vi "DAQ Assist.vi"(4 "timeout (s)":dbl=10.0 format="%0.2f", 5 "error in":errorcluster, 7 "stop (F)":bool, 10 "device name":tag="Mantis1_1Mod4") -> (14 "task out":refnum<k21>, 15 "data":dynamicdata(waveform), 18 "stopped":bool, 19 "error out":errorcluster)   [LabVIEW 2015]
doc: "Creates, edits, and runs tasks using NI-DAQmx. Refer to the NI-DAQmx Readme for a complete listing of devices NI-DAQmx supports.\n\nWhen you place this Express VI on the block diagram, the DAQ Assistant launches to create a new task. After you create a task, you can double-click the DAQ Assistant Express VI to edit that task. For continuous measurement or generation, place a while loop around the DAQ Assistant Express VI."
uses:
  <vilib>/DAQmx/read.llb/DAQmx Read.vi
  <vilib>/DAQmx/read.llb/DAQmx Read (Counter 1D U32 NChan 1Samp).vi
  <vilib>/DAQmx/miscellaneous.llb/DAQmx Fill In Error Info.vi
  <vilib>/DAQmx/create/channels.llb/DAQmx Create Channel (CI-Count Edges).vi
  <resource>/objmgr/daqmx.rc
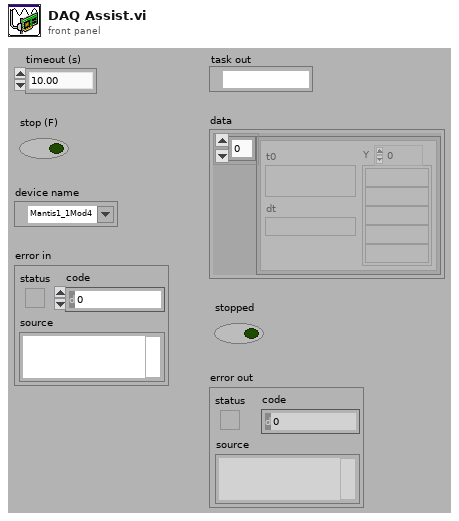
[diagram p1: front panel]
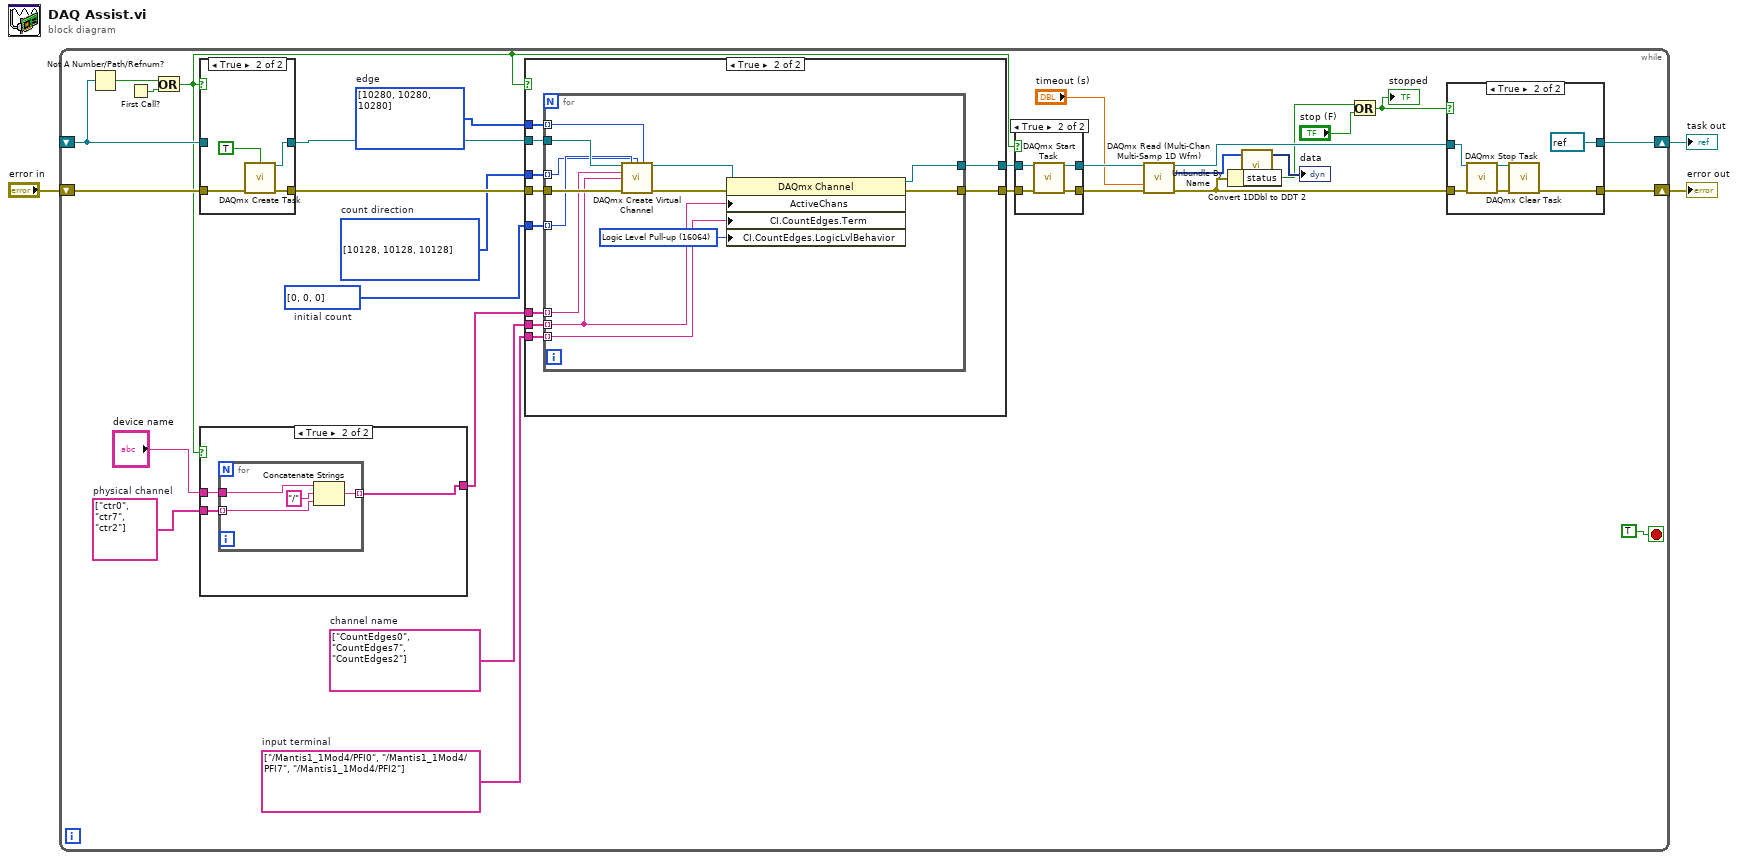
[diagram p0: block diagram]
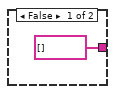
[diagram p5: hidden frame]
diagram:
  n1 = while {
    shift-right: [w10] -> w1
    shift-left: _ -> [w30]
    shift-right: [w8] -> w2
    shift-left: "error in" -> [w31]
    stop <- TRUE stop-if-true
    w19 = string[] ["/Mantis1_1Mod4/PFI0", "/Mantis1_1Mod4/PFI7", "/Mantis1_1Mod4/PFI2"]  # input terminal
    w22 = u32[] [0, 0, 0]  # initial count
    w23 = i32[] [10128, 10128, 10128] items=["Count Up"=10128, "Count Down"=10124, "Externally Controlled"=10326]  # count direction
    w24 = i32[] [10280, 10280, 10280] items=["Rising"=10280, "Falling"=10171]  # edge
    w20 = string[] ["CountEdges0", "CountEdges7", "CountEdges2"]  # channel name
    w27 = string[] ["ctr0", "ctr7", "ctr2"]  # physical channel
    n2 = Not A Number/Path/Refnum?(number/path/refnum=w30) -> (NaN/Path/Refnum?=w29:bool)
    n3 = First Call?() -> (First Call?: T/F=w32:bool)
    n4 = Or(x=w29, y=w32) -> (x .or. y?=w18:bool)
    n5 = case shown="True" w18 {
      tunnel: [w82 w86] -> w26
      tunnel: w30 -> [w82 _]
      tunnel: [w81 w85] -> w25
      tunnel: w31 -> [w81 w83]
      frame False {
      }
      frame True {
        n6 = call <vilib>:"DAQmx Create Task.vi"("auto cleanup"=TRUE, "error in"=w83) -> ("task out"=w86:refnum<k21>, "error out"=w85:errorcluster)  [unwired: 12 in]
      }
    }
    n7 = case shown="True" w18 {
      tunnel: [string[] [] w76] -> w21
      tunnel: "device name" -> [_ w75]
      tunnel: w27 -> [_ w74]
      frame False {
      }
      frame True {
        n8 = for {
          tunnel: [w80] -> w76 mode=indexing
          tunnel: w75 -> [w79]
          tunnel: w74 -> [w77] mode=indexing
          n9 = Concatenate Strings(w79, "/" ("string"), w77) -> (w80:string)
        }
      }
    }
    n10 = case shown="True" w18 {
      tunnel: [w49 w57] -> w17
      tunnel: w26 -> [w49 w59]
      tunnel: [w48 w56] -> w16
      tunnel: w25 -> [w48 w58]
      tunnel: w21 -> [_ w55]
      tunnel: w22 -> [_ w54]
      tunnel: w23 -> [_ w53]
      tunnel: w24 -> [_ w52]
      tunnel: w20 -> [_ w51]
      tunnel: w19 -> [_ w50]
      frame False {
      }
      frame True {
        n11 = for {
          tunnel: w59 -> [w72]
          tunnel: w58 -> [w71]
          tunnel: [w63] -> w57
          tunnel: [w65] -> w56
          tunnel: w55 -> [w69] mode=indexing
          tunnel: w54 -> [w68] mode=indexing
          tunnel: w53 -> [w67] mode=indexing
          tunnel: w52 -> [w66] mode=indexing
          tunnel: w51 -> [w62] mode=indexing
          tunnel: w50 -> [w61] mode=indexing
          w60 = 16064 items=["Logic Level Pull-up"=16064, "None"=10230] ("CI.CountEdges.LogicLvlBehavior")
          n12 = call-poly <vilib>:"DAQmx Create Virtual Channel.vi"("task in"=w72, "initial count"=w68, "count direction"=w67, "edge"=w66, "counter"=w69, "name to assign"=w62, "error in"=w71) -> ("task out"=w64:refnum<k21>, "error out"=w70:errorcluster)  [unwired: 7 in]
          n13 = property class="DAQmx Channel"(reference=w64, error in=w70, "ActiveChans"=w62, "CI.CountEdges.Term"=w61, "CI.CountEdges.LogicLvlBehavior"=w60) -> (reference out=w63:refnum<k21>, error out=w65:errorcluster)
        }
      }
    }
    n14 = case shown="True" w18 {
      tunnel: [w43 w46] -> w15
      tunnel: w17 -> [w43 w47]
      tunnel: [w42 w44] -> w14
      tunnel: w16 -> [w42 w45]
      frame False {
      }
      frame True {
        n15 = call <vilib>:"DAQmx Start Task.vi"("task/channels in"=w47, "error in"=w45) -> ("task out"=w46:refnum<k21>, "error out"=w44:errorcluster)  [unwired: 12 in]
      }
    }
    n16 = call-poly "DAQmx Read (Multi-Chan Multi-Samp 1D Wfm).vi"("task/channels in"=w15, "timeout"="timeout (s)", "error in"=w14) -> ("task out"=w9:refnum<k21>, "data"=w13:u32[], "error out"=w7:errorcluster)  [unwired: 10 in]
    n17 = Unbundle By Name(w7) -> ("status"=w6:bool)
    n18 = call <vilib>:"Convert 1DDbl to DDT 2.vi"("Array"=w13) -> ("Dynamic Data Type"=→"data":dynamicdata)  [unwired: 3 in]
    n19 = Or(x=w6, y="stop (F)") -> (x .or. y?=w4:bool)
    "stopped" <- w4
    n20 = case shown="True" w4 {
      tunnel: [w35 refnum<k21> refnum ("task in")] -> w10
      tunnel: w9 -> [w35 w41]
      tunnel: [w34 w38] -> w8
      tunnel: w7 -> [w34 w40]
      frame False {
      }
      frame True {
        n21 = call <vilib>:"DAQmx Stop Task.vi"("task/channels in"=w41, "error in"=w40) -> ("task out"=w37:refnum<k21>, "error out"=w39:errorcluster)  [unwired: 12 in]
        n22 = call <vilib>:"DAQmx Clear Task.vi"("task in"=w37, "error in"=w39) -> ("error out"=w38:errorcluster)  [unwired: 13 in]
      }
    }
  }
  "error out" <- w2
  "task out" <- w1
